vi "Reports.Report Config - Merge Legacy Config.vi"(9 "RemoteDataDir":path, 10 "LocalDataDir":path, 11 "RptCfg":T1[](array[typedef])) -> (1 "Changed":bool, 3 "RptCfg Out":T1[](array[typedef]))   [LabVIEW 2018]
uses:
  Report.Report File Config Item.ctl
  Report.Report File Type.ctl
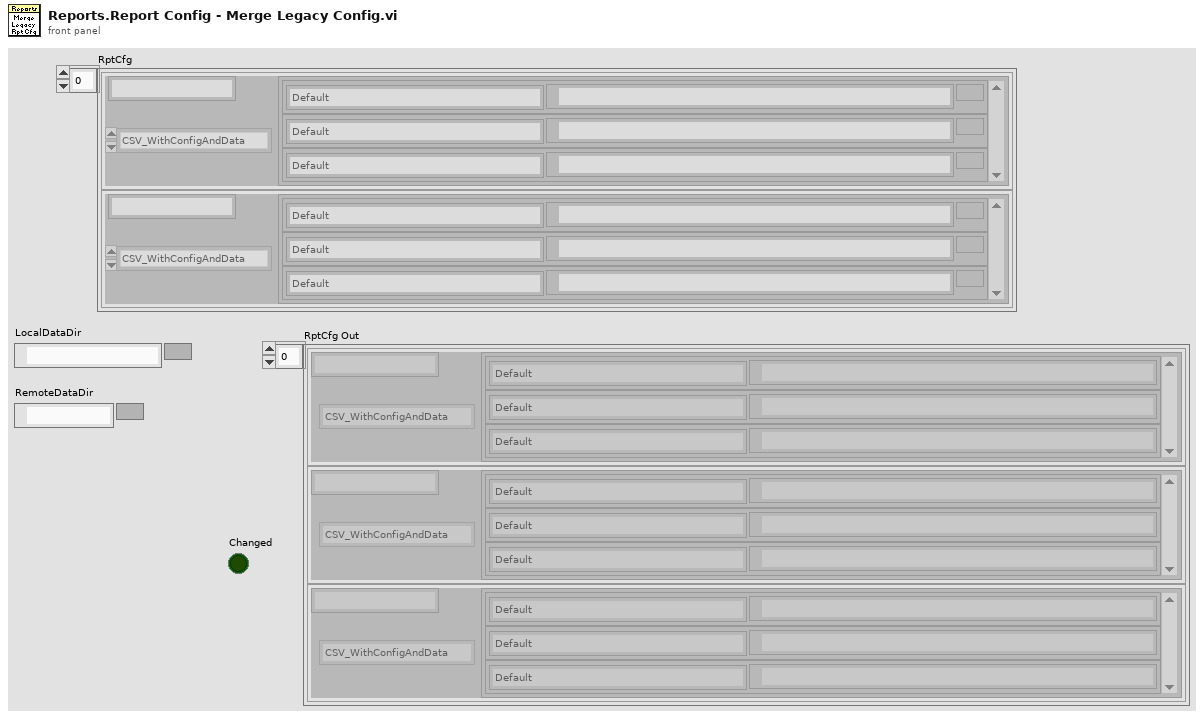
[diagram p1: front panel]
types:
  T1 = typedef "Report.Report File Config Item.ctl" = cluster{"Name":string, "Type":T2, "Seq_Dir":cluster{"Sequence":string, "Folder":path}[]}
  T2 = typedef "Report.Report File Type.ctl" = enum16{"CSV_WithConfigAndData", "CSV", "CSV_SummaryResult", "JSON", "JSON_WithFiles", "XLINK", "XLINK_ResultOnly", ""}
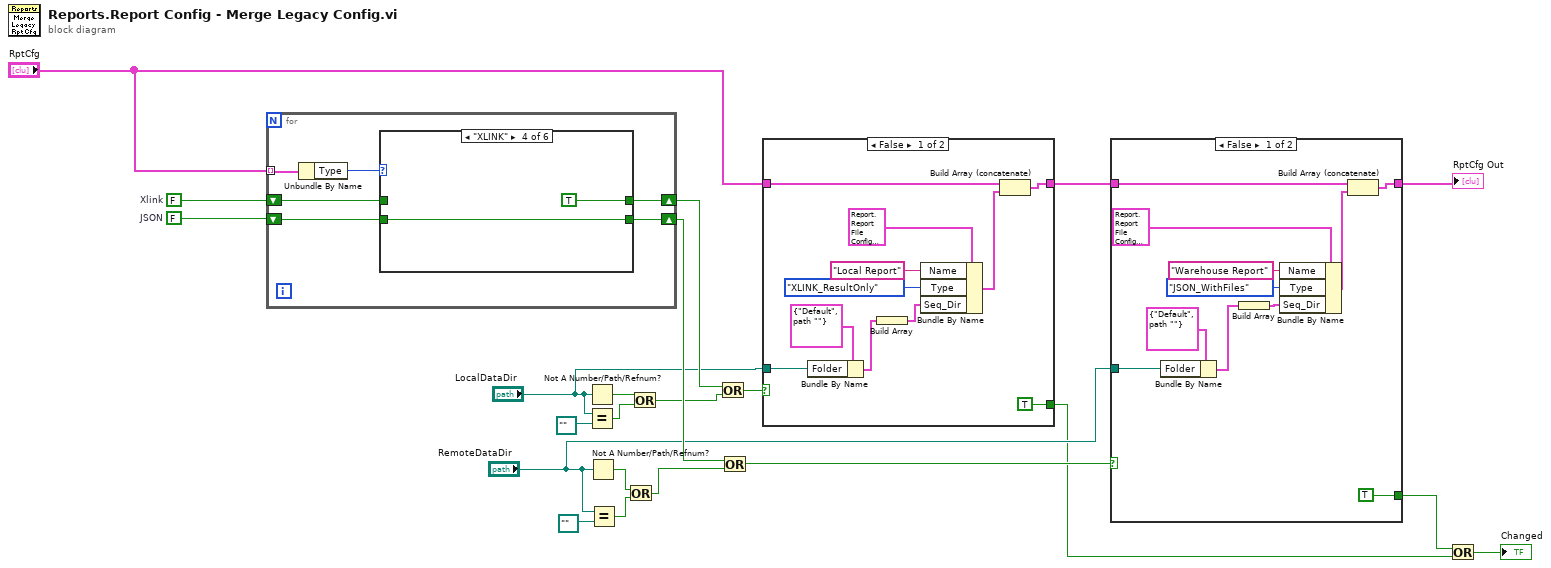
[diagram p0: block diagram]
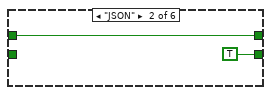
[diagram p5: hidden frame]
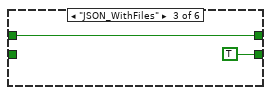
[diagram p6: hidden frame]
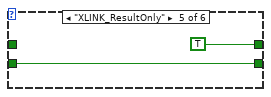
[diagram p7: hidden frame]
diagram:
  w21 = FALSE  # JSON
  w22 = FALSE  # Xlink
  n1 = for {
    tunnel: "RptCfg" -> [w28] mode=indexing
    shift-right: [w25] -> w19
    shift-left: w22 -> [w26]
    shift-right: [w23] -> w18
    shift-left: w21 -> [w24]
    n2 = Unbundle By Name(w28) -> ("Type"=w27:T2)
    n3 = case shown="\"XLINK\"" w27 {
      tunnel: w26 -> [w30 w32 w34 _ _ w40]
      tunnel: [w30 w32 w34 TRUE TRUE w40] -> w25
      tunnel: w24 -> [w29 _ _ w35 w37 w39]
      tunnel: [w29 TRUE TRUE w35 w37 w39] -> w23
      frame "CSV_WithConfigAndData" {
      }
      frame "JSON" {
      }
      frame "JSON_WithFiles" {
      }
      frame "XLINK" {
      }
      frame "XLINK_ResultOnly" {
      }
      frame "CSV", Default {
      }
    }
  }
  n4 = Not A Number/Path/Refnum?(number/path/refnum="LocalDataDir") -> (NaN/Path/Refnum?=w5:bool)
  n5 = Equal?(x="LocalDataDir", y=path "") -> (x = y?=w7:bool)
  n6 = Not A Number/Path/Refnum?(number/path/refnum="RemoteDataDir") -> (NaN/Path/Refnum?=w11:bool)
  n7 = Equal?(x="RemoteDataDir", y=path "") -> (x = y?=w10:bool)
  n8 = Or(x=w11, y=w10) -> (x .or. y?=w9:bool)
  n9 = Or(x=w5, y=w7) -> (x .or. y?=w4:bool)
  n10 = Or(x=w19, y=w4) -> (x .or. y?=w20:bool)
  n11 = Or(x=w18, y=w9) -> (x .or. y?=w15:bool)
  n12 = case shown="False" w20 {
    tunnel: "LocalDataDir" -> [w41 _]
    tunnel: "RptCfg" -> [w48 w52]
    tunnel: [w46 w52] -> w16
    tunnel: [TRUE _] -> w2
    frame False {
      n13 = Bundle By Name(cluster=cluster{"Sequence":string, "Folder":path} {"Sequence"="Default", "Folder"=path ""} ("Cluster"), "Folder"=w41) -> (w42:cluster{"Sequence":string, "Folder":path})
      n14 = Build Array(w42) -> (w44:cluster{"Sequence":string, "Folder":path}[])
      n15 = Bundle By Name(cluster=T1 {"Name"="", "Type"=enum."CSV_WithConfigAndData", "Seq_Dir"=[]}, "Name"="Local Report", "Type"=Report.Report_File_Type."XLINK_ResultOnly", "Seq_Dir"=w44) -> (w47:T1)
      n16 = Build Array (concatenate)(w48, w47) -> (w46:T1[])
    }
    frame True {
    }
  }
  n17 = case shown="False" w15 {
    tunnel: "RemoteDataDir" -> [w54 _]
    tunnel: w16 -> [w60 w64]
    tunnel: [w58 w64] -> w14
    tunnel: [TRUE _] -> w3
    frame False {
      n18 = Bundle By Name(cluster=cluster{"Sequence":string, "Folder":path} {"Sequence"="Default", "Folder"=path ""} ("Cluster"), "Folder"=w54) -> (w55:cluster{"Sequence":string, "Folder":path})
      n19 = Build Array(w55) -> (w53:cluster{"Sequence":string, "Folder":path}[])
      n20 = Bundle By Name(cluster=T1 {"Name"="", "Type"=enum."CSV_WithConfigAndData", "Seq_Dir"=[]}, "Name"="Warehouse Report", "Type"=Report.Report_File_Type."JSON_WithFiles", "Seq_Dir"=w53) -> (w59:T1)
      n21 = Build Array (concatenate)(w60, w59) -> (w58:T1[])
    }
    frame True {
    }
  }
  "RptCfg Out" <- w14
  n22 = Or(x=w3, y=w2) -> (x .or. y?=→"Changed":bool)
